vi "Tests.vi"() -> ()   [LabVIEW 2021, in "Tests.lvlib"]
uses:
  Tests.lvlib
  <vilib>/NI/Modbus Library/API/Wrapper/API Main.lvlib
  <vilib>/NI VeriStand/Custom Device API/Hardware Interface Driver VI Operation.ctl
  <vilib>/NI VeriStand/Custom Device API/Custom Device API.lvlib
  <vilib>/NI/Modbus Library/API/Master/Modbus Master.lvclass
  <vilib>/NI/Modbus Library/API/Wrapper/Create TCP Master.vi
  <vilib>/NI/Modbus Library/API/Wrapper/Create Serial Master.vi
  Shared/Controls/Interface Type.ctl
  Shared/Modbus Master Shared.lvlib
  Shared/Controls/Data Model/TCP Settings.ctl
  Shared/Controls/Data Model/Serial Settings.ctl
  System Explorer/SubVIs/Modbus Type.ctl
  Shared/Controls/Data Model/Channel.ctl
  Shared/Controls/Data Model/Input Channel Data.ctl
  Shared/Controls/Data Model/Output Channel Data.ctl
  <vilib>/NI VeriStand/Custom Device API/Custom Device Item Ref.ctl
  Shared/Controls/Data Model/Input References.ctl
  Shared/Device Info.ctl
panel:
  in  "Holding Registers":u16[](array[numeric])
  out "Input Registers":u16[](array[numeric])
  out "Discrete Inputs":bool[](array[boolean])
  in  "Coils":bool[](array[boolean])
  in  "stop":bool
  in  "Device Info":T1={"Name"="", "Unit ID"=0, "Interface Type"=enum."TCP Master", "TCP Settings"={"Address"="localhost", "Port"=502, "Timeout"=0}, "Serial Settings"={"VISA resource name"="", "baud rate"=9600, "parity (even)"=2, "flow control (none)"=0, "serial type"=enum."RTU", "Wire Mode"=-1}, "Inputs"={"Coils"=[{"Type"=enum."Coil", "Name"="coil0", "Mapping"=0, "Channel Array Index"=0}, {"Type"=enum."Coil", "Name"="coi1", "Mapping"=1, "Channel Array Index"=0}, {"Type"=enum."Coil", "Name"="coil2", "Mapping"=2, "Channel Array Index"=0}, {"Type"=enum."Coil", "Name"="coil3", "Mapping"=3, "Channel Array Index"=0}], "Discrete Inputs"=[{"Type"=enum."Discrete Input", "Name"="di0", "Mapping"=0, "Channel Array Index"=0}, {"Type"=enum."Discrete Input", "Name"="", "Mapping"=1, "Channel Array Index"=0}, {"Type"=enum."Discrete Input", "Name"="", "Mapping"=2, "Channel Array Index"=0}, {"Type"=enum."Discrete Input", "Name"="", "Mapping"=3, "Channel Array Index"=0}], "Input Registers"=[{"Type"=enum."Input Register", "Name"="", "Mapping"=0, "Channel Array Index"=0}, {"Type"=enum."Input Register", "Name"="", "Mapping"=1, "Channel Array Index"=0}, {"Type"=enum."Input Register", "Name"="", "Mapping"=2, "Channel Array Index"=0}, {"Type"=enum."Input Register", "Name"="", "Mapping"=3, "Channel Array Index"=0}], "Holding Registers"=[{"Type"=enum."Holding Register", "Name"="test 3", "Mapping"=0, "Channel Array Index"=0}]}, "Outputs"={"Coils"=[{"Type"=enum."Input Register", "Name"="", "Mapping"=0, "Channel Array Index"=0}, {"Type"=enum."Input Register", "Name"="", "Mapping"=1, "Channel Array Index"=0}, {"Type"=enum."Input Register", "Name"="", "Mapping"=2, "Channel Array Index"=0}, {"Type"=enum."Input Register", "Name"="", "Mapping"=3, "Channel Array Index"=0}], "Holding Registers"=[{"Type"=enum."Input Register", "Name"="", "Mapping"=0, "Channel Array Index"=0}, {"Type"=enum."Input Register", "Name"="", "Mapping"=1, "Channel Array Index"=0}, {"Type"=enum."Input Register", "Name"="", "Mapping"=2, "Channel Array Index"=0}, {"Type"=enum."Input Register", "Name"="", "Mapping"=3, "Channel Array Index"=0}]}, "References"={"Discrete Inputs"=[], "Input Registers"=[]}} {"References"."Input Registers" format="%.0x"; "References"."Discrete Inputs" format="%.0x"; "Serial Settings"."Wire Mode" items=["Unknown"=-1, "RS485/Wire4"=0, "RS485/Wire2-EchoDTR"=1, "RS485/Wire2-CtrlDTR"=2, "RS485/Wire2-Auto"=3, "RS232/DTE"=128, "RS232/DCE"=129, "RS232/AUTO"=130]; "Serial Settings"."parity (even)" items=["None", "Odd", "Even", "Mark", "Space"]; "Serial Settings"."flow control (none)" items=["None", "XON/XOFF", "RTS/CTS", "XON/XOFF & RTS/CTS", "DTR/DSR", "XON/XOFF & DTR/DSR"]}
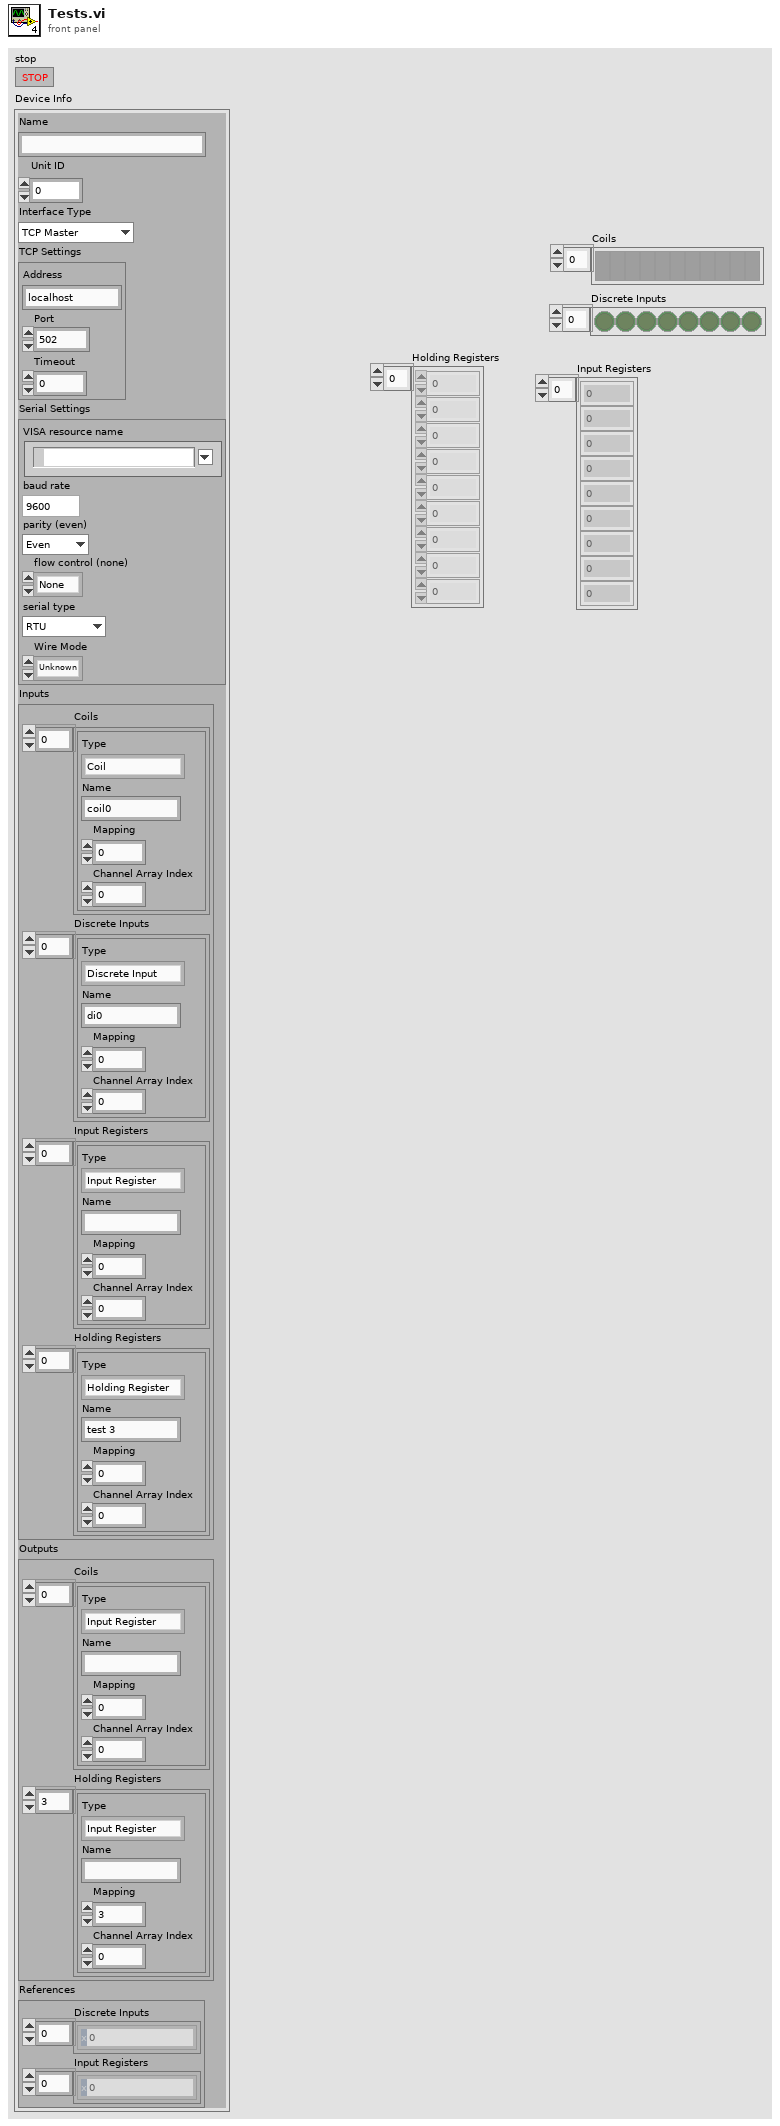
[diagram p1: front panel]
types:
  T1 = typedef "Modbus Master Shared.lvlib/Device Info.ctl" = cluster{"Name":string, "Unit ID":u8, "Interface Type":T2, "TCP Settings":T3, "Serial Settings":T4, "Inputs":T5, "Outputs":T8, "References":T9}
  T2 = typedef "Modbus Master Shared.lvlib/Interface Type.ctl" = enum16{"TCP Master", "Serial Master", "TCP Slave", "Serial Slave"}
  T3 = typedef "Modbus Master Shared.lvlib/TCP Settings.ctl" = cluster{"Address":string, "Port":u16, "Timeout":i32}
  T4 = typedef "Modbus Master Shared.lvlib/Serial Settings.ctl" = cluster{"VISA resource name":refnum<visa-resource-name>, "baud rate":u32, "parity (even)":u16, "flow control (none)":u16, "serial type":enum16{"RTU", "ASCII"}, "Wire Mode":i16}
  T5 = typedef "Modbus Master Shared.lvlib/Inputs.ctl" = cluster{"Coils":T6[], "Discrete Inputs":T6[], "Input Registers":T6[], "Holding Registers":T6[]}
  T6 = typedef "Modbus Master Shared.lvlib/Channel.ctl" = cluster{"Type":T7, "Name":string, "Mapping":u16, "Channel Array Index":i32}
  T7 = typedef "Modbus Master Shared.lvlib/Modbus Type.ctl" = enum16{"Coil", "Discrete Input", "Holding Register", "Input Register"}
  T8 = typedef "Modbus Master Shared.lvlib/Output Channel Data.ctl" = cluster{"Coils":T6[], "Holding Registers":T6[]}
  T9 = typedef "Modbus Master Shared.lvlib/Input References.ctl" = cluster{"Discrete Inputs":T10[], "Input Registers":T10[]}
  T10 = typedef "Custom Device API.lvlib/Custom Device Item Ref.ctl" = u64
  T11 = typedef "Custom Device API.lvlib/Hardware Interface Driver VI Operation.ctl" = enum16{"Initialize", "Start", "Read Data from HW", "Write Data to HW", "Close"}
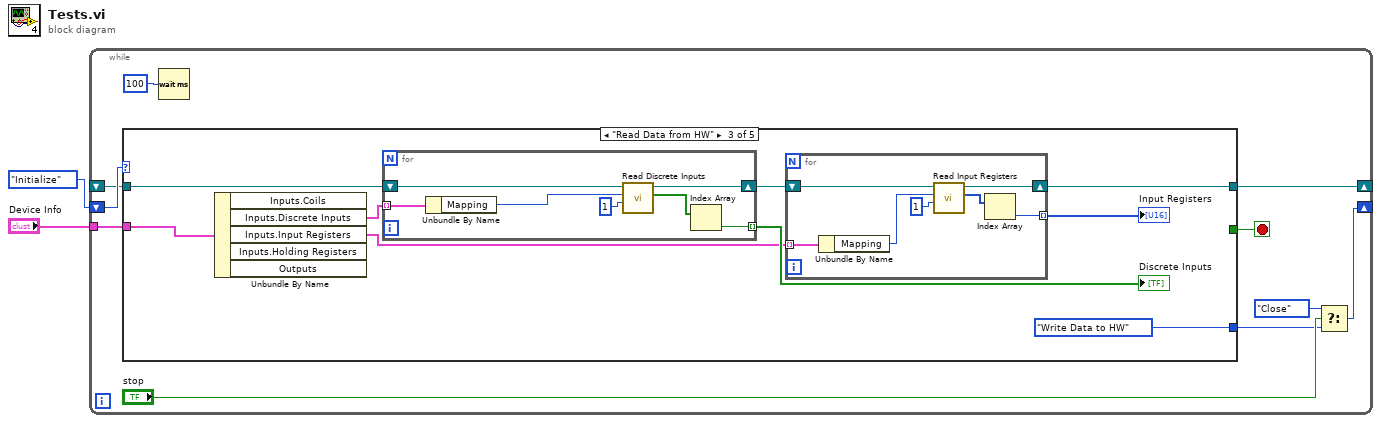
[diagram p0: block diagram]
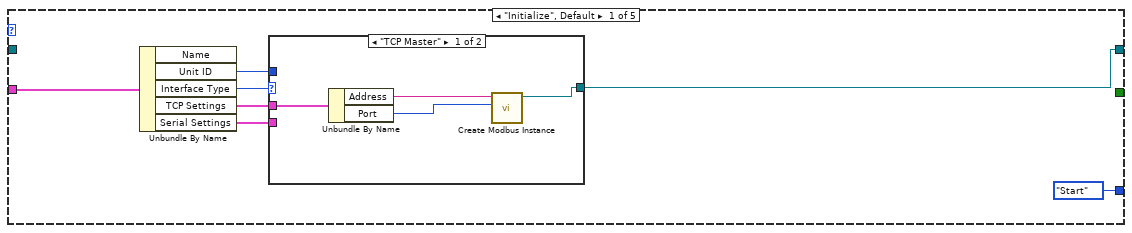
[diagram p2: hidden frame]
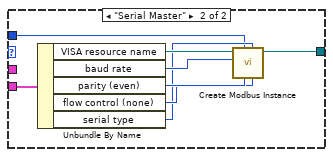
[diagram p3: hidden frame]
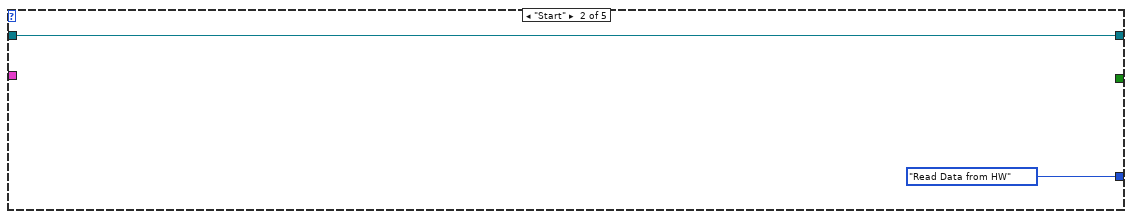
[diagram p4: hidden frame]
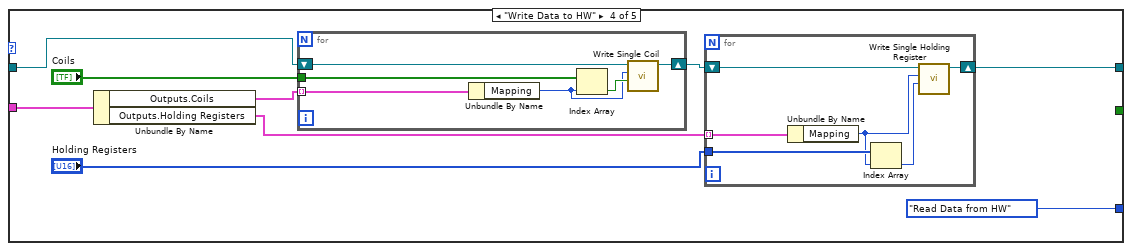
[diagram p5: hidden frame]
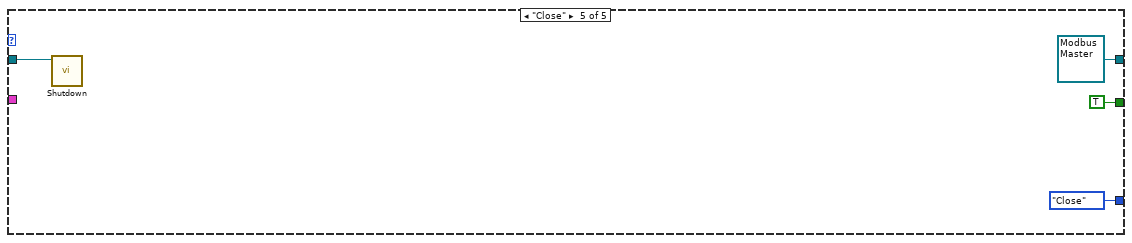
[diagram p6: hidden frame]
diagram:
  n1 = while {
    shift-right: [w4] -> _
    shift-left: Hardware_Interface_Driver_VI_Operation."Initialize" ("Operation") -> [w11]
    tunnel: "Device Info" -> [w10]
    shift-right: [w9] -> _
    shift-left: _ -> [w8]
    stop <- w3 stop-if-true
    n2 = case shown="\"Read Data from HW\"" w11 {
      tunnel: w10 -> [w19 _ w42 w62 _]
      tunnel: [w15 w33 w35 w57 refnum<class "Modbus Master.lvclass"> refnum ("Modbus master out")] -> w9
      tunnel: w8 -> [_ w33 w41 w64 w81]
      tunnel: [Hardware_Interface_Driver_VI_Operation."Start" ("Operation") Hardware_Interface_Driver_VI_Operation."Read Data from HW" ("Operation") Hardware_Interface_Driver_VI_Operation."Write Data to HW" ("Operation") Hardware_Interface_Driver_VI_Operation."Read Data from HW" ("Operation") Hardware_Interface_Driver_VI_Operation."Close" ("Operation")] -> w6
      tunnel: [_ _ _ _ TRUE] -> w3
      frame "Initialize", Default {
        n3 = Unbundle By Name(w19) -> ("Unit ID"=w14:u8, "Interface Type"=w18:T2, "TCP Settings"=w17:T3, "Serial Settings"=w16:T4)  [unwired: 1 out]
        n4 = case shown="\"TCP Master\"" w18 {
          tunnel: [w21 w26] -> w15
          tunnel: w17 -> [w20 _]
          tunnel: w16 -> [_ w25]
          tunnel: w14 -> [_ w24]
          frame "TCP Master" {
            n5 = Unbundle By Name(w20) -> ("Address"=w23:string, "Port"=w22:u16)
            n6 = call-poly <vilib>:"Create Modbus Instance.vi"("port (502)"=w22, "address"=w23) -> ("TCP master instance"=w21:refnum<class "Modbus Master.lvclass">)  [unwired: 8 in, 1 out]
          }
          frame "Serial Master" {
            n7 = Unbundle By Name(w25) -> ("VISA resource name"=w31:refnum<visa-resource-name>, "baud rate"=w30:u32, "parity (even)"=w29:u16, "flow control (none)"=w28:u16, "serial type"=w27:enum16{"RTU", "ASCII"})
            n8 = call-poly <vilib>:"Create Modbus Instance.vi"("flow control (none)"=w28, "serial type"=w27, "parity (even)"=w29, "unit ID"=w24, "baud rate"=w30, "VISA resource name"=w31) -> ("serial master instance"=w26:refnum<class "Modbus Master.lvclass">)  [unwired: 4 in, 1 out]
          }
        }
      }
      frame "Start" {
      }
      frame "Read Data from HW" {
        n9 = Unbundle By Name(w42) -> ("Inputs.Discrete Inputs"=w39:T6[], "Inputs.Input Registers"=w37:T6[])  [unwired: 3 out]
        n10 = for {
          tunnel: w39 -> [w56] mode=indexing
          shift-right: [w52] -> w36
          shift-left: w41 -> [w53]
          tunnel: [w50] -> w38 mode=indexing
          n11 = Unbundle By Name(w56) -> ("Mapping"=w55:u16)
          n12 = call-dynamic "Read Discrete Inputs.vi"("number of inputs"=u16 1, "starting address"=w55, "Modbus master in"=w53) -> ("discrete inputs"=w51:bool[], "Modbus master out"=w52:refnum<class "Modbus Master.lvclass">)  [unwired: 6 in, 1 out]
          n13 = Index Array(array=w51) -> (element=w50:bool)  [unwired: 1 in]
        }
        "Discrete Inputs" <- w38
        n14 = for {
          tunnel: w37 -> [w49] mode=indexing
          shift-right: [w46] -> w35
          shift-left: w36 -> [w47]
          tunnel: [w48] -> w34 mode=indexing
          n15 = Unbundle By Name(w49) -> ("Mapping"=w44:u16)
          n16 = call-dynamic "Read Input Registers.vi"("number of inputs"=u16 1, "starting address"=w44, "Modbus master in"=w47) -> ("register values"=w45:u16[], "Modbus master out"=w46:refnum<class "Modbus Master.lvclass">)  [unwired: 6 in, 1 out]
          n17 = Index Array(array=w45) -> (element=w48:u16)  [unwired: 1 in]
        }
        "Input Registers" <- w34
      }
      frame "Write Data to HW" {
        n18 = Unbundle By Name(w62) -> ("Outputs.Coils"=w61:T6[], "Outputs.Holding Registers"=w60:T6[])
        n19 = for {
          tunnel: w61 -> [w77] mode=indexing
          shift-right: [w75] -> w63
          shift-left: w64 -> [w76]
          tunnel: "Coils" -> [w74]
          n20 = Unbundle By Name(w77) -> ("Mapping"=w72:u16)
          n21 = Index Array(array=w74, index=w72) -> (element=w73:bool)
          n22 = call-dynamic "Write Single Coil.vi"("coil to write"=w73, "address"=w72, "Modbus master in"=w76) -> ("Modbus master out"=w75:refnum<class "Modbus Master.lvclass">)  [unwired: 7 in, 1 out]
        }
        n23 = for {
          tunnel: w60 -> [w71] mode=indexing
          shift-right: [w67] -> w57
          shift-left: w63 -> [w68]
          tunnel: "Holding Registers" -> [w69]
          n24 = Unbundle By Name(w71) -> ("Mapping"=w66:u16)
          n25 = Index Array(array=w69, index=w66) -> (element=w70:u16)
          n26 = call-dynamic "Write Single Holding Register.vi"("register to write"=w70, "address"=w66, "Modbus master in"=w68) -> ("Modbus master out"=w67:refnum<class "Modbus Master.lvclass">)  [unwired: 7 in, 1 out]
        }
      }
      frame "Close" {
        n27 = call-dynamic "Shutdown.vi"("Modbus master in"=w81) -> ()  [unwired: 10 in, 1 out]
      }
    }
    n28 = Wait (ms)(milliseconds to wait=u32 100) -> ()  [unwired: 1 out]
    n29 = Select(t=Hardware_Interface_Driver_VI_Operation."Close", s="stop", f=w6) -> (s? t:f=w4:T11)
  }
